vi "NI VeriStand - Get Alarm Data.vi"(8 "error in (no error)":errorcluster, 9 "timeout (ms)":u32=6000, 11 "Alarm in":T2) -> (0 "error out":errorcluster, 2 "Alarm Data":T1 {"Trip Value" format="%.2f"; "Delay" format="%.2f"; "Low Limit" format="%.2f"; "High Limit" format="%.2f"}, 3 "Alarm out":T2)   [LabVIEW 2020, in "NI_VS Alarm ExecutionAPI.lvlib"]
doc: "Returns high limit, low limit, corresponding procedure name, delay duration, trip value, priority, state, mode, group number, priority number, name, and full name information about the alarm you specify."
uses:
  <vilib>/NI VeriStand/Execution/Alarm/NI_VS Alarm ExecutionAPI.lvlib
  <vilib>/NI VeriStand/Execution/Alarm/AlarmAPI.ctl
  NationalInstruments.VeriStand.ClientAPI
  <vilib>/NI VeriStand/Execution/Alarm/AlarmInfo.ctl
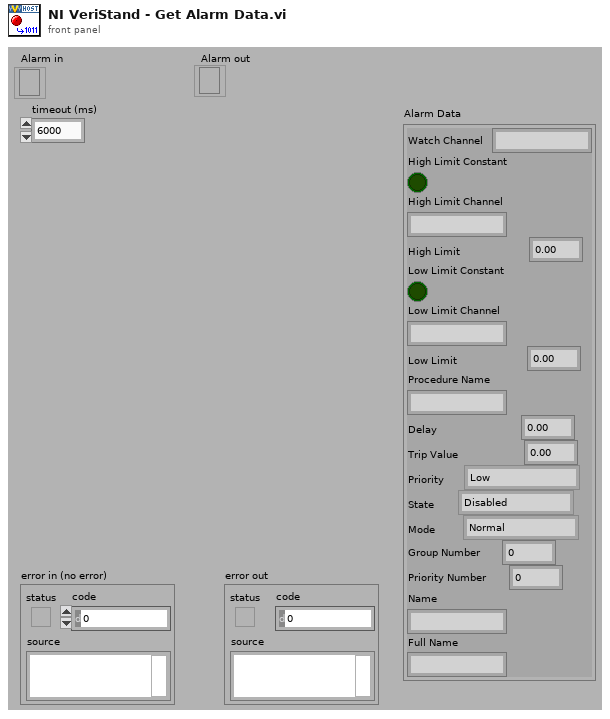
[diagram p1: front panel]
types:
  T1 = typedef "NI_VS Alarm ExecutionAPI.lvlib/AlarmInfo.ctl" = cluster{"Watch Channel":string, "High Limit Constant":bool, "High Limit Channel":string, "High Limit":dbl, "Low Limit Constant":bool, "Low Limit Channel":string, "Low Limit":dbl, "Procedure Name":string, "Delay":dbl, "Trip Value":dbl, "Priority":enum16{"Low", "Medium", "High"}, "State":enum16{"Disabled", "Enabled", "Tripped", "Delayed Trip", "Indicate"}, "Mode":enum16{"Normal", "Indicate Only"}, "Group Number":u32, "Priority Number":u32, "Name":string, "Full Name":string}
  T2 = typedef "NI_VS Alarm ExecutionAPI.lvlib/AlarmAPI.ctl" = refnum<k24>
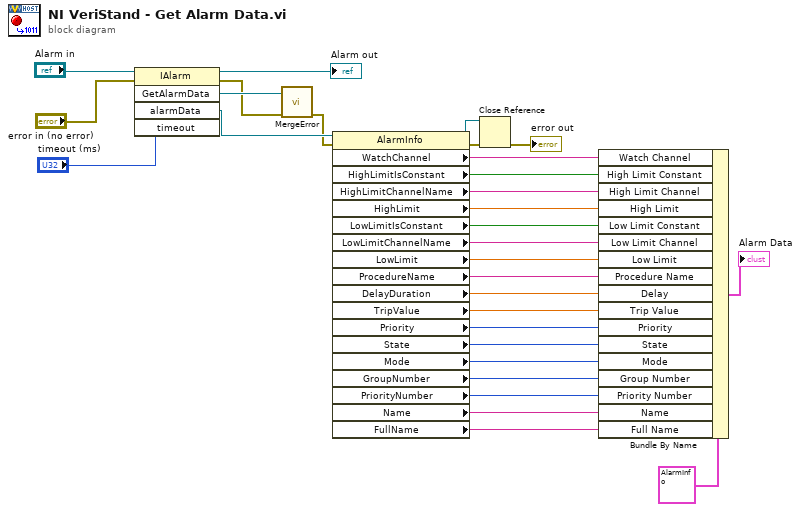
[diagram p0: block diagram]
diagram:
  n1 = invoke class="IAlarm" method="GetAlarmData"(reference="Alarm in", error in="error in (no error)", "timeout"="timeout (ms)") -> (reference out=→"Alarm out":T2, error out=w25:errorcluster, "GetAlarmData"=w28:refnum<k24>, "alarmData"=w26:refnum<k24>)  [unwired: 2 in, 1 out]
  n2 = call <vilib>:"MergeError.vi"("error in (no error)"=w25, "Error"=w28) -> ("error out"=w24:errorcluster)  [unwired: 9 out]
  n3 = property class="AlarmInfo"(reference=w26, error in=w24) -> (reference out=w22:refnum<k24>, error out=w23:errorcluster, "WatchChannel"=w19:string, "HighLimitIsConstant"=w18:bool, "HighLimitChannelName"=w17:string, "HighLimit"=w16:dbl, "LowLimitIsConstant"=w15:bool, "LowLimitChannelName"=w14:string, "LowLimit"=w13:dbl, "ProcedureName"=w12:string, "DelayDuration"=w11:dbl, "TripValue"=w10:dbl, "Priority"=w9:u8, "State"=w8:u8, "Mode"=w7:u8, "GroupNumber"=w4:u32, "PriorityNumber"=w3:u32, "Name"=w2:string, "FullName"=w1:string)
  n4 = Close Reference(reference=w22, error in (no error)=w23) -> (error out=→"error out":errorcluster)
  n5 = Bundle By Name(cluster=T1 {"Watch Channel"="", "High Limit Constant"=FALSE, "High Limit Channel"="", "High Limit"=0.0, "Low Limit Constant"=FALSE, "Low Limit Channel"="", "Low Limit"=0.0, "Procedure Name"="", "Delay"=0.0, "Trip Value"=0.0, "Priority"=enum."Low", "State"=enum."Disabled", "Mode"=enum."Normal", "Group Number"=0, "Priority Number"=0, "Name"="", "Full Name"=""} ("AlarmInfo"), "Watch Channel"=w19, "High Limit Constant"=w18, "High Limit Channel"=w17, "High Limit"=w16, "Low Limit Constant"=w15, "Low Limit Channel"=w14, "Low Limit"=w13, "Procedure Name"=w12, "Delay"=w11, "Trip Value"=w10, "Priority"=w9, "State"=w8, "Mode"=w7, "Group Number"=w4, "Priority Number"=w3, "Name"=w2, "Full Name"=w1) -> (→"Alarm Data":T1)
